vi "Preview_Build.vi"(8 "error in (no error)":errorcluster, 11 "Build in":refnum<class "AB_Build.lvclass">) -> (0 "error out":errorcluster, 1 "GeneratedFiles":path[](array[path]), 3 "Build out":refnum<class "AB_Build.lvclass">, 4 "GeneratedFileGUIDs":string[](array[string]), 5 "OutputDirectory":path)   [LabVIEW 2020, in "AB_Build.lvclass"]
uses:
  <vilib>/AppBuilder/AB_Classes/Build/AB_Build.lvclass
  <vilib>/AppBuilder/AB_Classes/Build/AB_Build.lvclass/AB_Build.ctl
  <vilib>/AppBuilder/AB_Source_Inclusion.ctl
  <resource>/Framework/Providers/Common/provcom_StringGlobals.vi
  <vilib>/AppBuilder/AB_Classes/Destination/AB_Destination.lvclass
  <vilib>/AppBuilder/AB_Classes/Source/AB_Source.lvclass
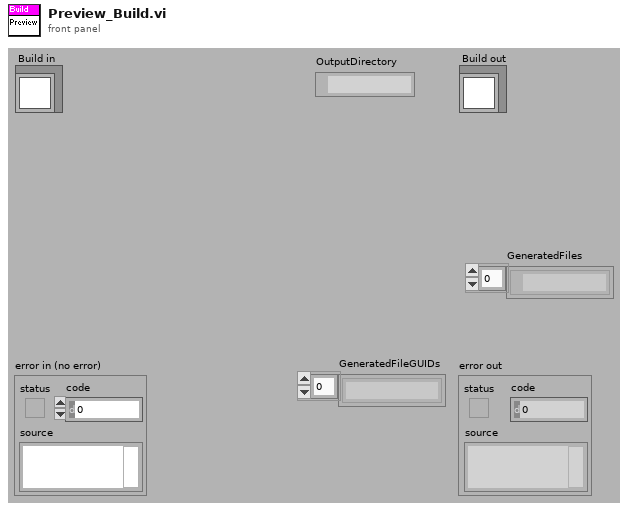
[diagram p1: front panel]
types:
  T1 = typedef "AB_Source_Inclusion.ctl" = enum16{"IncludeIfReferenced", "Include", "Exclude", "TopLevel"}
  T2 = typedef "mxLvBuildError.ctl" = refnum<user-event>
  T3 = typedef "AB_Destination.ctl" = cluster{"destName":string, "path":path, "libraryName":string, "preserveHierarchy":bool, "eng_inBuild":bool, "eng_libraryReference":refnum<vi>, "eng_restictAddToNewLibrary":bool}
  T4 = typedef "AB_Source.ctl" = cluster{"path":path, "itemID":string, "parentIndex":i32, "sourceInclusion":T1, "destinationIndex":i32, "properties":T5[], "newName":string, "lvfile":bool, "valid":bool, "eng_inBuild":bool, "eng_isNonVILink":bool, "Amalgamation":bool, "Amalgamation Piece":bool, "eng_delimitedName":string, "preventRename":bool}
  T5 = typedef "AB_Source_Properties.ctl" = cluster{"sourcePropertyType":T6, "value":variant}
  T6 = typedef "AB_Source_Property_Type.ctl" = enum16{"Remove block diagram", "Remove front panel", "Password", "Window has title bar", "Show menu bar", "Show vertical scroll bar", "Show horizontal scroll bar", "Show toolbar", "Show Abort button", "Show fp when called", "Window behavior", "Allow user to close window", "Window run-time position", "Run when opened", "Allow debugging", "Auto error handling", "Generate guard code", "Use stack variables", "Expression folding", "Integer only", "Inline subVI"}
  T7 = typedef "ItemRef.ctl" = u64
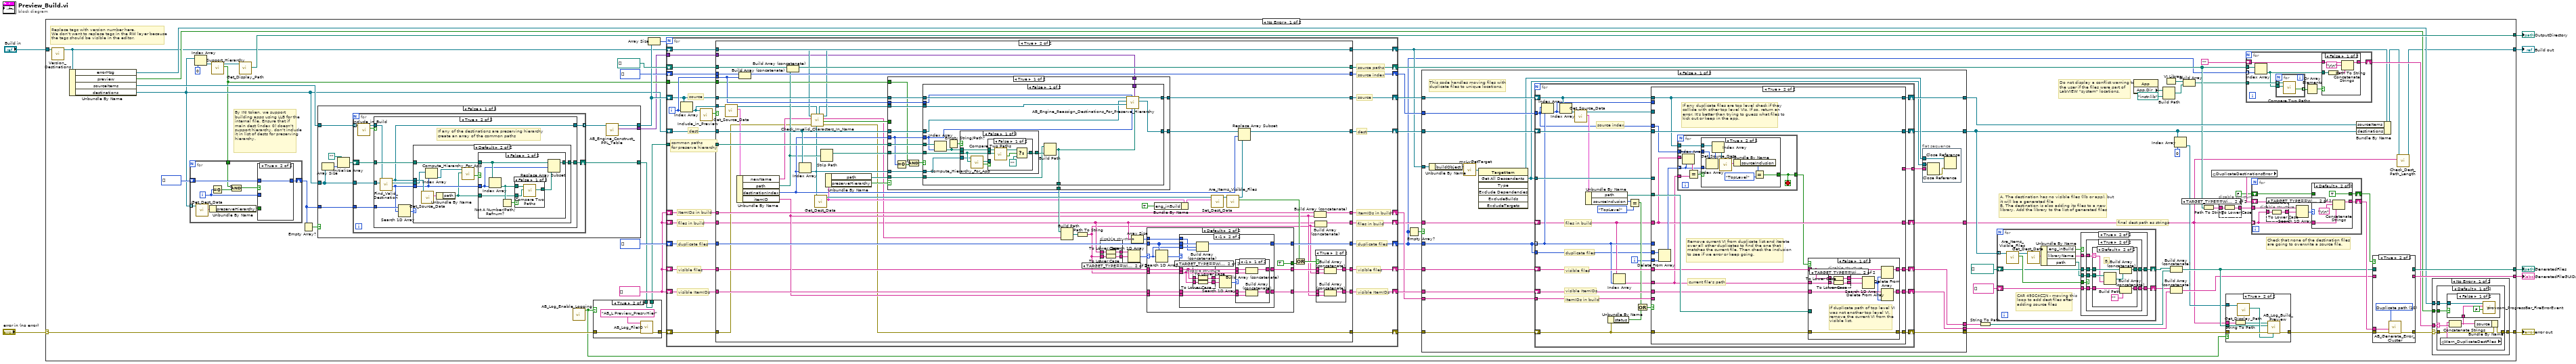
[diagram p0: block diagram]
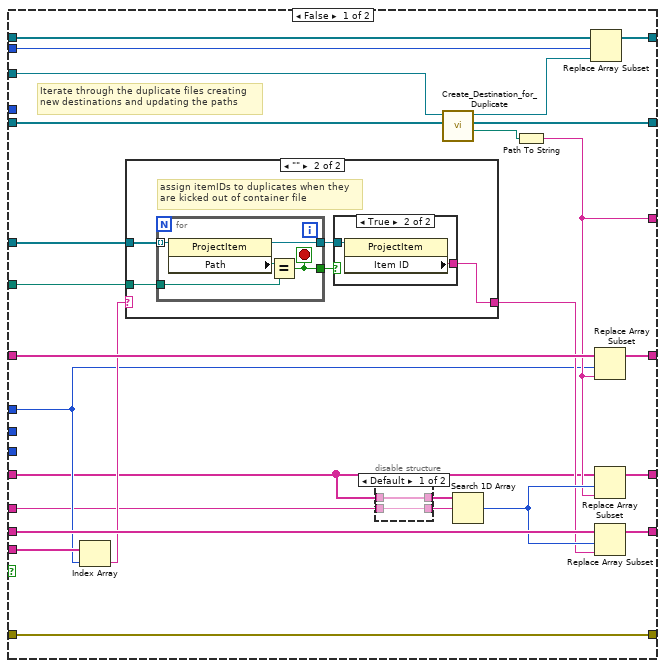
[diagram p3: hidden frame]
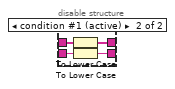
[diagram p4: hidden frame]
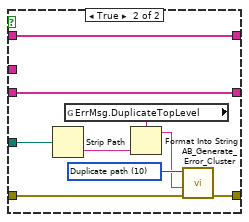
[diagram p9: hidden frame]
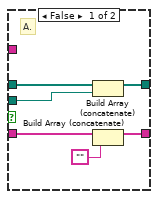
[diagram p13: hidden frame]
diagram:
  n1 = case shown="No Error" "error in (no error)" {
    selector: "error in (no error)" -> [w31 w663]
    tunnel: [w49 w663] -> w6
    tunnel: [w16 w662] -> w4
    tunnel: "Build in" -> [w14 w662]
    tunnel: [w56 _] -> w3
    tunnel: [w55 _] -> w2
    tunnel: [w57 _] -> w1
    frame No Error {
      w37 = string[] []
      # "Replace tags with version number here.\nWe don't want to replace tags in the RW layer because\nthe tags should be visible in the editor."
      # "final dest path as strings"
      # "Do not display a conflict warning to the user if the files were part of LabVIEW \"system\" locations."
      # "By INI token, we support building apps using LLB for the internal file. Ensure that if main dest (index 0) doesn't support hierarchy, don't include it in list of dests for preserving hierarchy."
      # "A. The destination has no visible files (llb or app), but it will be a generated file\nB. The destination is also adding its files to a new library. Add the library to the list of generated files"
      # "Check that none of the destination files are going to overwrite a source file."
      n2 = call <vilib>:"Version_Destinations.vi"("Class in"=w14) -> ("Class out"=w13:refnum<class "AB_Build.lvclass">)  [unwired: 9 in, 1 out]
      n3 = Unbundle By Name(w13) -> ("errorMsg"=w52:T2, "preview"=w50:bool, "sourceItems"=w69:refnum<class "AB_Source.lvclass">[], "destinations"=w35:refnum<class "AB_Destination.lvclass">[])
      n4 = Index Array(array=w35, index=0) -> (element=w34:refnum<class "AB_Destination.lvclass">)
      n5 = call-dynamic "Support_Hierarchy.vi"("AB_Destination in"=w34) -> ("support hierarchy"=w32:bool, "AB_Destination out"=w33:refnum<class "AB_Destination.lvclass">)  [unwired: 1 in, 8 out]
      n6 = for {
        tunnel: w35 -> [w648] mode=indexing
        shift-right: [w650] -> w70
        shift-left: i32[] [] -> [w649]
        tunnel: w32 -> [w645]
        i -> [w647]
        n7 = call <vilib>:"Get_Dest_Data.vi"("Class in"=w648) -> ("destName"=w652:T3)  [unwired: 1 in, 9 out]
        n8 = Unbundle By Name(w652) -> ("preserveHierarchy"=w651:bool)
        n9 = Equal To 0?(x=w647) -> (x = 0?=w646:bool)
        n10 = Compound Arithmetic op=AND(invert w645, w646) -> (w644:bool)
        n11 = case shown="True" w644 {
          tunnel: w651 -> [w656 _]
          tunnel: [w655 w661] -> w650
          tunnel: w649 -> [w654 w661]
          tunnel: w647 -> [w653 _]
          frame False {
            n12 = case shown="False" w656 {
              tunnel: w653 -> [_ w660]
              tunnel: [w657 w659] -> w655
              tunnel: w654 -> [w657 w658]
              frame False {
              }
              frame True {
                n13 = Build Array (concatenate)(w658, w660) -> (w659:i32[])
              }
            }
          }
          frame True {
          }
        }
      }
      n14 = call-dynamic "Get_Display_Path.vi"("AB_Destination in"=w33) -> ("displayPath"=w57:path)  [unwired: 1 in, 9 out]
      n15 = Empty Array?(array=w70) -> (empty?=w71:bool)
      n16 = case shown="False" w71 {
        tunnel: w35 -> [w338 w386]
        tunnel: w69 -> [w341 w388]
        tunnel: w70 -> [w340 _]
        tunnel: [w339 _] -> w29
        tunnel: [w337 w387] -> w68
        tunnel: [w335 _] -> w10
        frame False {
          n17 = Array Size(array=w338) -> (size(s)=w344:i32)
          n18 = Initialize Array(path "", w344) -> (w342:path[])
          n19 = for {
            shift-right: [w351] -> w339
            shift-left: w342 -> [w350]
            tunnel: w341 -> [w347] mode=indexing
            tunnel: w340 -> [w352]
            tunnel: [w348] -> w336 mode=indexing
            tunnel: w338 -> [w349]
            n20 = call-dynamic "Include_in_Build.vi"("AB_Source in"=w347) -> ("includeInBuild"=w345:bool, "AB_Source out"=w346:refnum<class "AB_Source.lvclass">)  [unwired: 1 in, 8 out]
            n21 = case shown="True" w345 {
              tunnel: w352 -> [_ w363]
              tunnel: [w353 w361] -> w351
              tunnel: w350 -> [w353 w360]
              tunnel: w346 -> [w354 w359]
              tunnel: w349 -> [_ w358]
              tunnel: [w354 w356] -> w348
              frame False {
              }
              frame True {
                # "If any of the destinations are preserving hierarchy\ncreate an array of the common paths"
                n22 = call <vilib>:"Find_Valid_Destination.vi"("Destinations in"=w358, "AB_Source in"=w359) -> ("destinationIndex"=w357:i32, "Destinations out"=w355:refnum<class "AB_Destination.lvclass">[], "AB_Source out"=w356:refnum<class "AB_Source.lvclass">)  [unwired: 1 in, 6 out]
                n23 = Search 1D Array(1D array=w363, element=w357) -> (index of element=w362:i32)  [unwired: 1 out]
                n24 = case shown="Default" w362 {
                  tunnel: [w364 w372] -> w361
                  tunnel: w360 -> [w364 w373]
                  tunnel: w357 -> [_ w367]
                  tunnel: w356 -> [_ w370]
                  tunnel: w355 -> [_ w368]
                  frame -1 {
                  }
                  frame Default {
                    n25 = call <vilib>:"Get_Source_Data.vi"("Class in"=w370) -> ("data"=w371:T4)  [unwired: 1 in, 9 out]
                    n26 = Index Array(array=w368, index=w367) -> (element=w366:refnum<class "AB_Destination.lvclass">)
                    n27 = Unbundle By Name(w371) -> ("path"=w365:path)
                    n28 = call-dynamic "Compute_Hierarchy_For_App.vi"("sourcePath"=w365, "AB_Destination in"=w366) -> ("relative to AppDir"=w369:bool)  [unwired: 1 in, 8 out]
                    n29 = case shown="False" w369 {
                      tunnel: w373 -> [w378 w385]
                      tunnel: [w377 w385] -> w372
                      tunnel: w367 -> [w375 _]
                      tunnel: w365 -> [w374 _]
                      frame False {
                        n30 = Index Array(array=w378, index=w375) -> (element=w379:path)
                        n31 = Not A Number/Path/Refnum?(number/path/refnum=w379) -> (NaN/Path/Refnum?=w380:bool)
                        n32 = case shown="False" w380 {
                          tunnel: w379 -> [w383 _]
                          tunnel: w374 -> [w382 w384]
                          tunnel: [w381 w384] -> w376
                          frame False {
                            n33 = call <vilib>:"Compare Two Paths.vi"("Path 2"=w382, "Path 1"=w383) -> ("Common Path"=w381:path)  [unwired: 1 in, 8 out]
                          }
                          frame True {
                          }
                        }
                        n34 = Replace Array Subset(array=w378, new element=w376, index=w375) -> (w377:path[])
                      }
                      frame True {
                        # "If source file path is relative to LabVIEW dir (when dest is an app), don't include LabVIEW's dir in the list of common paths. This reduces the depth of the hierarchy we compute.\nDo standard hierarchy calculations for other dests."
                      }
                    }
                  }
                }
              }
            }
          }
          n35 = call <vilib>:"AB_Engine_Construct_PPL_Table.vi"("sources in"=w336) -> ("PPL Table"=w335:variant, "sources out"=w337:refnum<class "AB_Source.lvclass">[])  [unwired: 8 in, 1 out]
        }
        frame True {
          n36 = for {
            tunnel: w388 -> [w391] mode=indexing
            tunnel: [w392] -> w387 mode=indexing
            tunnel: w386 -> [w393]
            n37 = call-dynamic "Include_in_Build.vi"("AB_Source in"=w391) -> ("includeInBuild"=w389:bool, "AB_Source out"=w390:refnum<class "AB_Source.lvclass">)  [unwired: 1 in, 8 out]
            n38 = case shown="True" w389 {
              tunnel: w390 -> [w394 w397]
              tunnel: w393 -> [_ w396]
              tunnel: [w394 w395] -> w392
              frame False {
              }
              frame True {
                # "Still have to validate destinations to make sure nonVI files aren't targeted into an llb/zip and amalgamation files aren't targeted into an llb"
                n39 = call <vilib>:"Find_Valid_Destination.vi"("Destinations in"=w396, "AB_Source in"=w397) -> ("AB_Source out"=w395:refnum<class "AB_Source.lvclass">)  [unwired: 1 in, 8 out]
              }
            }
          }
        }
      }
      n40 = call <vilib>:"AB_Log_Enable_Logging.vi"() -> ("log?"=w30:bool)  [unwired: 2 in, 9 out]
      n41 = case shown="True" w30 {
        tunnel: w31 -> [w246 w249]
        tunnel: [w246 w248] -> w21
        tunnel: w29 -> [w245 w247]
        tunnel: [w245 w247] -> w28
        frame False {
        }
        frame True {
          n42 = call <vilib>:"AB_Log_FileIO.vi"("error in (no error)"=w249, "newSection"="AB_L Preview_PresrvHier" ("data")) -> ("error out"=w248:errorcluster)  [unwired: 3 in, 6 out]
        }
      }
      n43 = Array Size(array=w68) -> (size(s)=w79:i32)
      n44 = for {
        N: w79 -> [_]
        shift-right: [w431] -> w65
        shift-left: w68 -> [w432]
        shift-right: [w449] -> w47
        shift-left: w37 -> [w450]
        shift-right: [w448] -> w48
        shift-left: w37 -> [w447]
        shift-right: [w445] -> w66
        shift-left: w35 -> [w446]
        shift-right: [w443] -> w27
        shift-left: path[] [] -> [w444]
        tunnel: w28 -> [w442]
        shift-right: [w441] -> w12
        shift-left: i32[] [] -> [w440]
        shift-right: [w438] -> w63
        shift-left: i32[] [] -> [w439]
        shift-right: [w435] -> w60
        shift-left: w37 -> [w436]
        shift-right: [w434] -> w59
        shift-left: w37 -> [w433]
        tunnel: w32 -> [w428]
        shift-right: [w426] -> w20
        shift-left: w21 -> [w427]
        shift-right: [w424] -> _
        shift-left: w13 -> [w425]
        tunnel: w10 -> [w423]
        i -> [w437]
        # "source index"
        # "dest"
        # "source"
        # "dest"
        # "visible ItemIDs"
        # "ItemIDs in build"
        # "visible ItemIDs"
        # "ItemIDs in build"
        # "visible files"
        # "duplicate files"
        # "source paths"
        # "files in build"
        # "visible files"
        # "duplicate files"
        # "common paths\nfor preserve hierarchy"
        # "source"
        # "files in build"
        n45 = Index Array(array=w432, index=w437) -> (element=w429:refnum<class "AB_Source.lvclass">)
        n46 = call-dynamic "Include_in_Preview.vi"("AB_Source in"=w429) -> ("includeInPreview"=w430:bool)  [unwired: 9 in, 1 out]
        n47 = case shown="True" w430 {
          tunnel: w437 -> [_ w486]
          tunnel: w450 -> [w460 w478]
          tunnel: [w460 w505] -> w449
          tunnel: [w461 w520] -> w448
          tunnel: w447 -> [w461 w465]
          tunnel: w429 -> [_ w484]
          tunnel: w446 -> [w459 w492]
          tunnel: [w459 w518] -> w445
          tunnel: w444 -> [w458 w516]
          tunnel: [w458 w487] -> w443
          tunnel: w442 -> [_ w510]
          tunnel: [w457 w507] -> w441
          tunnel: w440 -> [w457 w506]
          tunnel: w439 -> [w456 w499]
          tunnel: [w456 w488] -> w438
          tunnel: w436 -> [w455 w498]
          tunnel: [w455 w494] -> w435
          tunnel: [w454 w497] -> w434
          tunnel: w433 -> [w454 w496]
          tunnel: w432 -> [w453 w490]
          tunnel: [w453 w489] -> w431
          tunnel: w428 -> [_ w477]
          tunnel: w427 -> [w452 w474]
          tunnel: [w452 w473] -> w426
          tunnel: w425 -> [w451 w472]
          tunnel: [w451 w471] -> w424
          tunnel: w423 -> [_ w466]
          frame False {
          }
          frame True {
            n48 = call <vilib>:"Get_Source_Data.vi"("Class in"=w484) -> ("data"=w485:T4, "Class out"=w470:refnum<class "AB_Source.lvclass">)  [unwired: 1 in, 8 out]
            n49 = Unbundle By Name(w485) -> ("newName"=w475:string, "path"=w481:path, "destinationIndex"=w482:i32, "itemID"=w493:string)
            n50 = Build Array (concatenate)(w499, w486) -> (w488:i32[])
            n51 = Build Array (concatenate)(w516, w481) -> (w487:path[])
            n52 = Index Array(array=w492, index=w482) -> (element=w476:refnum<class "AB_Destination.lvclass">)
            n53 = call-dynamic "Check_Invalid_Characters_In_Name.vi"("AB_Destination in"=w476, "AB_Source in"=w470, "error in (no error)"=w474, "file name in"=w475, "Build in"=w472) -> ("error out"=w473:errorcluster, "updated"=w468:bool, "file name out"=w467:string, "Build out"=w471:refnum<class "AB_Build.lvclass">, "AB_Source out"=w469:refnum<class "AB_Source.lvclass">)  [unwired: 1 in, 1 out]
            n54 = call <vilib>:"Get_Dest_Data.vi"("Class in"=w476) -> ("destName"=w483:T3, "Class out"=w513:refnum<class "AB_Destination.lvclass">)  [unwired: 1 in, 8 out]
            n55 = Strip Path(path=w481) -> (stripped path=w509:path)  [unwired: 1 out]
            n56 = Unbundle By Name(w483) -> ("path"=w479:path, "preserveHierarchy"=w511:bool)
            n57 = case shown="True" w511 {
              tunnel: w510 -> [w550 _]
              tunnel: w509 -> [w549 _]
              tunnel: [w547 w590] -> w508
              tunnel: w479 -> [w548 w590]
              tunnel: w482 -> [w539 _]
              tunnel: w492 -> [w546 w591]
              tunnel: [w545 w591] -> w491
              tunnel: w490 -> [w544 w588]
              tunnel: [w543 w587] -> w489
              tunnel: w486 -> [w542 w589]
              tunnel: w469 -> [w541 w586]
              tunnel: w477 -> [w538 _]
              tunnel: w476 -> [w536 _]
              tunnel: w468 -> [_ w585]
              tunnel: w466 -> [w535 _]
              frame True {
                n58 = Equal To 0?(x=w539) -> (x = 0?=w540:bool)
                n59 = Compound Arithmetic op=AND(invert w538, w540) -> (w537:bool)
                n60 = case shown="False" w537 {
                  tunnel: w550 -> [w566 _]
                  tunnel: w549 -> [w564 _]
                  tunnel: w548 -> [w562 w582]
                  tunnel: [w558 w582] -> w547
                  tunnel: w546 -> [w555 w583]
                  tunnel: [w554 w583] -> w545
                  tunnel: w544 -> [w557 w584]
                  tunnel: [w553 w584] -> w543
                  tunnel: w542 -> [w552 _]
                  tunnel: w541 -> [w556 _]
                  tunnel: w539 -> [w559 _]
                  tunnel: w536 -> [w560 _]
                  tunnel: w535 -> [w551 _]
                  frame False {
                    n61 = Index Array(array=w566, index=w559) -> (element=w561:path)
                    n62 = Empty String/Path?(string/path=w561) -> (empty?=w565:bool)
                    n63 = case shown="False" w565 {
                      tunnel: w564 -> [w568 w581]
                      tunnel: w561 -> [w572 _]
                      tunnel: [w571 w580] -> w563
                      tunnel: w560 -> [w567 _]
                      frame False {
                        n64 = call-dynamic "Compute_Hierarchy_For_App.vi"("sourcePath"=w568, "AB_Destination in"=w567) -> ("relative to AppDir"=w570:bool, "destinationPath"=w569:path)  [unwired: 1 in, 7 out]
                        n65 = case shown="False" w570 {
                          tunnel: w568 -> [w578 _]
                          tunnel: w572 -> [w577 _]
                          tunnel: [w573 w579] -> w571
                          tunnel: w569 -> [_ w579]
                          frame False {
                            n66 = call <vilib>:"Compare Two Paths.vi"("Path 2"=w578, "Path 1"=w577) -> ("Path 2 Relative to Path 1?"=w574:bool, "Relative Path from 1 to 2"=w575:path)  [unwired: 1 in, 7 out]
                            n67 = Select(t=w575, s=w574, f=path "") -> (s? t:f=w573:path)
                          }
                          frame True {
                          }
                        }
                      }
                      frame True {
                        n68 = call <vilib>:"AB_Convert_To_Relative_Path.vi"("absolute path"=w581) -> ("relative path"=w580:path)  [unwired: 10 in]
                      }
                    }
                    n69 = Build Path(base path=w562, name or relative path=w563) -> (appended path=w558:path)
                    n70 = call <vilib>:"AB_Engine_Reassign_Destinations_For_Preserve_Hierarchy.vi"("newPath"=w558, "PPL Table"=w551, "parentIndex in"=w559, "source index"=w552, "source"=w556, "destinations in"=w555, "sources in"=w557) -> ("destination out"=w554:refnum<class "AB_Destination.lvclass">[], "sources out"=w553:refnum<class "AB_Source.lvclass">[])  [unwired: 2 in, 1 out]
                  }
                  frame True {
                    # "By INI token, we support building apps using LLB for the internal file. Ensure that if main dest (index 0) doesn't support hierarchy, don't try preserving hierarchy since we can't."
                  }
                }
              }
              frame False {
                n71 = case shown="True" w585 {
                  tunnel: w589 -> [_ w596]
                  tunnel: w588 -> [w592 w595]
                  tunnel: [w592 w594] -> w587
                  tunnel: w586 -> [_ w593]
                  frame False {
                  }
                  frame True {
                    # "If filename was updated, update the value in the source array."
                    n72 = Replace Array Subset(array=w595, new element=w593, index=w596) -> (w594:refnum<class "AB_Source.lvclass">[])
                  }
                }
              }
            }
            n73 = Build Path(base path=w508, name or relative path=w467) -> (appended path=w480:path)
            n74 = Path To String(path=w480) -> (string=w463:string)
            n75 = disable-structure shown="TARGET_TYPE==Windows" {
              disable-tunnel: w465 -> [w522 w525]
              disable-tunnel: [w522 w526] -> w464
              disable-tunnel: w463 -> [w521 w524]
              disable-tunnel: [w521 w523] -> w462
              frame condition #0 {
              }
              frame condition #1 (active) {
                n76 = To Lower Case(string=w525) -> (all lower case string=w526:string[])
                n77 = To Lower Case(string=w524) -> (all lower case string=w523:string)
              }
            }
            n78 = Search 1D Array(1D array=w464, element=w462) -> (index of element=w519:i32)  [unwired: 1 out]
            n79 = Array Size(array=w465) -> (size(s)=w500:i32)
            n80 = case shown="Default" w519 {
              selector: w519 -> [_ w608]
              tunnel: w500 -> [_ w603]
              tunnel: [w599 w611] -> w507
              tunnel: w506 -> [w599 w610]
              tunnel: [_ TRUE] -> w502
              tunnel: w478 -> [w598 w606]
              tunnel: w463 -> [_ w605]
              tunnel: [w598 w604] -> w501
              tunnel: w498 -> [w597 w602]
              tunnel: w493 -> [_ w601]
              tunnel: [w597 w600] -> w495
              frame -1 {
              }
              frame Default {
                n81 = Search 1D Array(1D array=w610, element=w608) -> (index of element=w609:i32)  [unwired: 1 out]
                n82 = case shown="-1" w609 {
                  tunnel: w603 -> [w613 w624]
                  tunnel: [w616 w629] -> w611
                  tunnel: w610 -> [w615 w628]
                  tunnel: w608 -> [_ w627]
                  tunnel: w606 -> [w614 w620]
                  tunnel: w605 -> [_ w618]
                  tunnel: [w614 w625] -> w604
                  tunnel: w602 -> [w612 w623]
                  tunnel: w601 -> [_ w622]
                  tunnel: [w612 w621] -> w600
                  frame Default {
                    n83 = Build Array (concatenate)(w615, w613) -> (w616:i32[])
                  }
                  frame -1 {
                    n84 = disable-structure shown="TARGET_TYPE==Windows" {
                      disable-tunnel: w620 -> [w631 w634]
                      disable-tunnel: [w631 w635] -> w619
                      disable-tunnel: w618 -> [w630 w633]
                      disable-tunnel: [w630 w632] -> w617
                      frame condition #0 {
                      }
                      frame condition #1 (active) {
                        n85 = To Lower Case(string=w634) -> (all lower case string=w635:string[])
                        n86 = To Lower Case(string=w633) -> (all lower case string=w632:string)
                      }
                    }
                    n87 = Build Array (concatenate)(w628, w627, w624) -> (w629:i32[])
                    n88 = Search 1D Array(1D array=w619, element=w617) -> (index of element=w626:i32)  [unwired: 1 out]
                    n89 = case shown="-1" w626 {
                      tunnel: w620 -> [w641 w643]
                      tunnel: w618 -> [w640 _]
                      tunnel: [w639 w643] -> w625
                      tunnel: w623 -> [w638 w642]
                      tunnel: w622 -> [w637 _]
                      tunnel: [w636 w642] -> w621
                      frame -1 {
                        n90 = Build Array (concatenate)(w641, w640) -> (w639:string[])
                        n91 = Build Array (concatenate)(w638, w637) -> (w636:string[])
                      }
                      frame Default {
                      }
                    }
                  }
                }
              }
            }
            n92 = Bundle By Name(cluster=w483, "eng_inBuild"=TRUE) -> (w512:T3)
            n93 = call <vilib>:"Set_Dest_Data.vi"("destName"=w512, "Class in"=w513) -> ("Class out"=w514:refnum<class "AB_Destination.lvclass">)  [unwired: 1 in, 8 out]
            n94 = call-dynamic "Are_Items_Visible_Files.vi"("AB_Destination in"=w514) -> ("itemsVisibleFiles"=w504:bool, "AB_Destination out"=w517:refnum<class "AB_Destination.lvclass">)  [unwired: 1 in, 8 out]
            n95 = Replace Array Subset(array=w491, new element=w517, index=w482) -> (w518:refnum<class "AB_Destination.lvclass">[])
            n96 = Or(x=w504, y=w502) -> (x .or. y?=w503:bool)
            n97 = Build Array (concatenate)(w496, w493) -> (w497:string[])
            n98 = Build Array (concatenate)(w465, w463) -> (w520:string[])
            n99 = case shown="True" w503 {
              tunnel: w501 -> [w528 w534]
              tunnel: [w528 w533] -> w505
              tunnel: w463 -> [_ w532]
              tunnel: w495 -> [w527 w531]
              tunnel: [w527 w530] -> w494
              tunnel: w493 -> [_ w529]
              frame False {
              }
              frame True {
                n100 = Build Array (concatenate)(w534, w532) -> (w533:string[])
                n101 = Build Array (concatenate)(w531, w529) -> (w530:string[])
              }
            }
          }
        }
      }
      n102 = Empty Array?(array=w12) -> (empty?=w11:bool)
      n103 = case shown="False" w11 {
        tunnel: w66 -> [w103 w243]
        tunnel: w65 -> [w102 w244]
        tunnel: w63 -> [w101 _]
        tunnel: [w100 w244] -> w62
        tunnel: w60 -> [w99 w239]
        tunnel: w59 -> [w98 _]
        tunnel: w48 -> [w97 w242]
        tunnel: w47 -> [w96 w241]
        tunnel: [w95 w241] -> w46
        tunnel: [w94 w239] -> w38
        tunnel: [w93 w240] -> w36
        tunnel: w20 -> [w89 w240]
        tunnel: [w88 w243] -> w18
        tunnel: [w87 w242] -> w15
        tunnel: w13 -> [w86 _]
        tunnel: w12 -> [w83 _]
        frame False {
          # "This code handles moving files with duplicate files to unique locations."
          n104 = Unbundle By Name(w86) -> ("buildObject"=w84:T7)
          n105 = call <resource>:"mxLvGetTarget.vi"("Item"=w84) -> ("Target"=w85:refnum<vi>)  [unwired: 1 in, 2 out]
          n106 = invoke class="TargetItem" method="Get All Descendents"(reference=w85) -> (reference out=w91:refnum<vi>, "All Descendents"=w92:refnum<vi>[])  [unwired: 6 in, 5 out]
          n107 = for {
            shift-right: [w132] -> w87
            shift-left: w97 -> [w111]
            shift-right: [w136] -> w88
            shift-left: w103 -> [w135]
            shift-right: [w134] -> w100
            shift-left: w102 -> [w133]
            shift-right: [w131] -> w95
            shift-left: w96 -> [w130]
            tunnel: w83 -> [w112] mode=indexing
            tunnel: w101 -> [w107]
            shift-right: [w128] -> w94
            shift-left: w99 -> [w127]
            tunnel: w98 -> [w126]
            tunnel: w92 -> [w125]
            tunnel: [w122] -> w90
            shift-right: [w121] -> w93
            shift-left: w89 -> [w119]
            tunnel: w83 -> [w108]
            i -> [w109]
            # "duplicate files"
            # "source index"
            # "visible ItemIDs"
            # "visible files"
            # "files in build"
            # "ItemIDs in build"
            n108 = Index Array(array=w107, index=w112) -> (element=w129:i32)
            n109 = Index Array(array=w133, index=w129) -> (element=w124:refnum<class "AB_Source.lvclass">)
            n110 = call <vilib>:"Get_Source_Data.vi"("Class in"=w124) -> ("data"=w120:T4, "Class out"=w123:refnum<class "AB_Source.lvclass">)  [unwired: 1 in, 8 out]
            n111 = Unbundle By Name(w120) -> ("path"=w113:path, "sourceInclusion"=w116:T1)
            n112 = Unbundle By Name(w119) -> ("status"=w117:bool)
            n113 = Index Array(array=w111, index=w112) -> (element=w110:string)
            n114 = Equal?(x=w116, y=AB_Source_Inclusion."TopLevel") -> (x = y?=w114:bool)
            n115 = Or(x=w114, y=w117) -> (x .or. y?=w118:bool)
            n116 = case shown="True" w118 {
              tunnel: [w162 w197] -> w136
              tunnel: w135 -> [w161 w197]
              tunnel: [w160 w186] -> w134
              tunnel: w133 -> [w159 w186]
              tunnel: [w157 w185] -> w132
              tunnel: w111 -> [w156 w185]
              tunnel: [w155 w191] -> w131
              tunnel: w130 -> [w140 w192]
              tunnel: w129 -> [w154 _]
              tunnel: [w153 w190] -> w128
              tunnel: w127 -> [w152 w193]
              tunnel: w126 -> [w151 _]
              tunnel: w112 -> [w142 _]
              tunnel: w125 -> [w148 _]
              tunnel: w123 -> [w147 _]
              tunnel: [w144 _] -> w122
              tunnel: w119 -> [w143 w195]
              tunnel: [w143 w196] -> w121
              tunnel: w113 -> [w141 w194]
              tunnel: w110 -> [w138 w183]
              tunnel: w109 -> [_ w188]
              tunnel: w108 -> [_ w189]
              tunnel: w107 -> [_ w184]
              frame False {
                # "Iterate through the duplicate files creating\nnew destinations and updating the paths"
                n117 = Index Array(array=w151, index=w142) -> (element=w146:string)
                n118 = case shown="\"\"" w146 {
                  selector: w146 -> [w169 _]
                  tunnel: w148 -> [_ w174]
                  tunnel: [w169 w171] -> w145
                  tunnel: w141 -> [_ w170]
                  frame Default {
                  }
                  frame "" {
                    # "assign itemIDs to duplicates when they are kicked out of container file"
                    n119 = for {
                      tunnel: w174 -> [w181] mode=indexing
                      tunnel: w170 -> [w177]
                      tunnel: [w179] -> w172
                      tunnel: [w178] -> w173
                      stop <- w178 stop-if-true
                      n120 = property class="ProjectItem"(reference=w181) -> (reference out=w179:refnum<vi>, "Path"=w180:path)  [unwired: 1 in, 1 out]
                      n121 = Equal?(x=w180, y=w177) -> (x = y?=w178:bool)
                    }
                    n122 = case shown="True" w173 {
                      tunnel: w172 -> [_ w176]
                      tunnel: [_ w175] -> w171
                      frame False {
                      }
                      frame True {
                        n123 = property class="ProjectItem"(reference=w176) -> ("Item ID"=w175:string)  [unwired: 1 in, 2 out]
                      }
                    }
                  }
                }
                n124 = disable-structure shown="Default" {
                  disable-tunnel: w140 -> [w164 w167]
                  disable-tunnel: [w164 w168] -> w139
                  disable-tunnel: w138 -> [w163 w166]
                  disable-tunnel: [w163 w165] -> w137
                  frame condition #0 {
                  }
                  frame condition #1 (active) {
                    n125 = To Lower Case(string=w167) -> (all lower case string=w168:string[])
                    n126 = To Lower Case(string=w166) -> (all lower case string=w165:string)
                  }
                }
                n127 = call-dynamic "Create_Destination_for_Duplicate.vi"("Destinations in"=w161, "AB_Source in"=w147) -> ("newPath"=w149:path, "Destinations out"=w162:refnum<class "AB_Destination.lvclass">[], "AB_Source out"=w158:refnum<class "AB_Source.lvclass">)  [unwired: 2 in, 5 out]
                n128 = Search 1D Array(1D array=w139, element=w137) -> (index of element=w150:i32)  [unwired: 1 out]
                n129 = Path To String(path=w149) -> (string=w144:string)
                n130 = Replace Array Subset(array=w159, new element=w158, index=w154) -> (w160:refnum<class "AB_Source.lvclass">[])
                n131 = Replace Array Subset(array=w156, new element=w144, index=w142) -> (w157:string[])
                n132 = Replace Array Subset(array=w140, new element=w144, index=w150) -> (w155:string[])
                n133 = Replace Array Subset(array=w152, new element=w145, index=w150) -> (w153:string[])
              }
              frame True {
                # "Remove current VI from duplicate list and iterate over all other duplicates to find the one that matches the current file. Then check the inclusion to see if we error or keep going."
                # "current file's path"
                # "If any duplicate files are top level check if they collide with other top level VIs. If so, return an error. It's better than trying to guess what files to kick out or keep in the app."
                n134 = Delete From Array(array=w189, index=w188) -> (array with subset deleted=w187:i32[])  [unwired: 1 in, 1 out]
                n135 = for {
                  tunnel: w187 -> [w200] mode=indexing
                  tunnel: w186 -> [w199]
                  tunnel: w185 -> [w205]
                  tunnel: w184 -> [w204]
                  tunnel: w183 -> [w202]
                  tunnel: [w198] -> w182
                  stop <- w198 stop-if-true
                  n136 = Index Array(array=w205, index=w200) -> (element=w203:string)
                  n137 = Equal?(x=w203, y=w202) -> (x = y?=w201:bool)
                  n138 = case shown="True" w201 {
                    tunnel: w204 -> [_ w214]
                    tunnel: w200 -> [_ w213]
                    tunnel: w199 -> [_ w211]
                    tunnel: [_ w206] -> w198
                    frame False {
                    }
                    frame True {
                      n139 = Index Array(array=w214, index=w213) -> (element=w212:i32)
                      n140 = Index Array(array=w211, index=w212) -> (element=w210:refnum<class "AB_Source.lvclass">)
                      n141 = call <vilib>:"Get_Source_Data.vi"("Class in"=w210) -> ("data"=w209:T4)  [unwired: 1 in, 9 out]
                      n142 = Unbundle By Name(w209) -> ("sourceInclusion"=w208:T1)
                      n143 = Equal?(x=w208, y=AB_Source_Inclusion."TopLevel") -> (x = y?=w206:bool)
                    }
                  }
                }
                n144 = case shown="False" w182 {
                  tunnel: [w223 w238] -> w196
                  tunnel: w195 -> [w223 w237]
                  tunnel: w194 -> [_ w235]
                  tunnel: w193 -> [w221 w230]
                  tunnel: w192 -> [w218 w231]
                  tunnel: [w222 w231] -> w191
                  tunnel: [w220 w230] -> w190
                  tunnel: w183 -> [w216 _]
                  frame False {
                    # "If duplicate path of top level VI was not another top level VI, remove the current VI from the visible list."
                    n145 = disable-structure shown="TARGET_TYPE==Windows" {
                      disable-tunnel: w218 -> [w225 w228]
                      disable-tunnel: [w225 w229] -> w217
                      disable-tunnel: w216 -> [w224 w227]
                      disable-tunnel: [w224 w226] -> w215
                      frame condition #0 {
                      }
                      frame condition #1 (active) {
                        n146 = To Lower Case(string=w228) -> (all lower case string=w229:string[])
                        n147 = To Lower Case(string=w227) -> (all lower case string=w226:string)
                      }
                    }
                    n148 = Search 1D Array(1D array=w217, element=w215) -> (index of element=w219:i32)  [unwired: 1 out]
                    n149 = Delete From Array(array=w218, index=w219) -> (array with subset deleted=w222:string[])  [unwired: 1 in, 1 out]
                    n150 = Delete From Array(array=w221, index=w219) -> (array with subset deleted=w220:string[])  [unwired: 1 in, 1 out]
                  }
                  frame True {
                    w236 = 10 items=["No error", "Argument error", "Memory is full", "Out of zone", "End of file", "File already open", "Generic file I/O error", "File not found", "File permission error", "Disk is full", "Duplicate path", "Too many files open", "System feature not enabled", "Resource file not found", "Cannot add resource", "Resource not found", "Image not found", "Image memory error", "Pen does not exist", "Config type invalid", "Config token not found", "Config parse error", "Config memory error", "Bad external code format", "Bad external code offset", "External code not present", "Null window", "Destroy window error", "Null menu", "Print aborted", "Bad print record", "Print driver error", "Windows error during printing", "Memory error during printing", "Print dialog error", "Generic print error", "Invalid device refnum", "Device not found", "Device parameter error", "Device unit error", "Cannot open device", "Device call aborted", "Generic error", "Cancelled by user", "Object ID too low", "Object ID too high", "Object not in heap", "Unknown heap", "Unknown object (invalid DefProc)", "Unknown object (DefProc not in table)", "Message out of range", "Invalid (null) method", "Unknown message", "Manager call not supported", "Bad address", "Network operation in progress", "Network operation timed out", "Connection is busy", "Network attribute not supported", "Network error", "Address in use", "System out of memory", "Connection aborted", "Connection refused", "Not connected", "Already connected", "Connection closed", "Initialization error (interapplication manager)", "Bad occurrence", "Wait on unbound occurrence handler", "Occurrence queue overflow", "Datalog type conflict", "Unused", "Unrecognized type (interapplication manager)", "Memory corrupt", "Failed to make temporary DLL", "Old CIN version", "Drag socket not found", "Failed to load drop-object", "Failed to register OLE object", "Failed to release OLE object", "Format specifier type mismatch", "Unknown format specifier", "Too few format specifiers", "Too many format specifiers", "Scan failed", "Newer CIN version", "Error converting to variant", "Runtime menu error", "Password tampered", "Variant attribute not found", "Incompatible variant data type", "Event data is not available", "Event Store is not present", "Occurrence is not found", "Event Queue is not created", "Event info is not available in the type library", "Refnum passed is NULL", "Error retrieving Class GUID", "Error retrieving CoClass GUID", "Error retrieving TypeLib GUID.", "Bad built application magic bytes.", "Specific driver is different from the specific driver associated with the Logical Name.", "There is no session opened to the class driver.", "Max Error", "MAX - Error with config objects", "MAX - Error loading configuration", "MAX - Group not supported", "Singlecast connections can not send to multicast addresses.", "Multicast connections can not send to singlecast addresses.", "Specified IP address not in multicast address range.", "Attempt to write to read-only multicast connection.", "Attempt to read from write-only multicast connection.", "The buffer used to receive a datagram was smaller than the datagram itself"] ("Code")
                    n151 = Strip Path(path=w235) -> (name=w233:string)  [unwired: 1 out]
                    n152 = global read "provcom_StringGlobals.vi" "ErrMsg.DuplicateTopLevel"() -> (w234:string)
                    n153 = Format Into String(format string=w234, w233) -> (resulting string=w232:string)  [unwired: 2 in, 1 out]
                    n154 = call <vilib>:"AB_Generate_Error_Cluster.vi"("error in (no error)"=w237, "Additional Message"=w232, "Code"=w236) -> ("error out"=w238:errorcluster)  [unwired: 1 in, 7 out]
                  }
                }
              }
            }
          }
          n155 = flat-sequence {
            tunnel: w92 -> [w106]
            tunnel: w91 -> [w105]
            tunnel: w90 -> [_]
            frame #0 {
              n156 = Close Reference(reference=w106) -> (error out=w104:errorcluster)  [unwired: 1 in]
              n157 = Close Reference(reference=w105, error in (no error)=w104) -> ()  [unwired: 1 out]
            }
          }
        }
        frame True {
        }
      }
      n158 = String To Path(string=w46) -> (path=w45:path[])
      n159 = for {
        tunnel: w18 -> [w261] mode=indexing
        shift-right: [w258] -> w44
        shift-left: path[] [] -> [w259]
        shift-right: [w253] -> w40
        shift-left: string[] [] -> [w252]
        # "CAR 49SC4CZN - moving this loop to add dest files after adding source files"
        n160 = call-dynamic "Are_Items_Visible_Files.vi"("AB_Destination in"=w261) -> ("itemsVisibleFiles"=w260:bool, "AB_Destination out"=w256:refnum<class "AB_Destination.lvclass">)  [unwired: 1 in, 8 out]
        n161 = call <vilib>:"Get_Dest_Data.vi"("Class in"=w256) -> ("destName"=w257:T3)  [unwired: 1 in, 9 out]
        n162 = Unbundle By Name(w257) -> ("eng_inBuild"=w251:bool, "libraryName"=w255:string, "path"=w254:path)
        n163 = case shown="True" w251 {
          tunnel: w260 -> [_ w270]
          tunnel: w259 -> [w263 w269]
          tunnel: [w263 w268] -> w258
          tunnel: w255 -> [_ w267]
          tunnel: w254 -> [_ w266]
          tunnel: [w262 w265] -> w253
          tunnel: w252 -> [w262 w264]
          frame False {
            # "Dest not participating in build"
          }
          frame True {
            n164 = case shown="True" w270 {
              tunnel: w269 -> [w276 w282]
              tunnel: [w275 w281] -> w268
              tunnel: w266 -> [w274 w279]
              tunnel: w267 -> [_ w280]
              tunnel: [w271 w278] -> w265
              tunnel: w264 -> [w272 w277]
              frame False {
                # "A."
                n165 = Build Array (concatenate)(w276, w274) -> (w275:path[])
                n166 = Build Array (concatenate)(w272, "") -> (w271:string[])
              }
              frame True {
                n167 = case shown="Default" w280 {
                  selector: w280 -> [_ w289]
                  tunnel: w282 -> [w284 w292]
                  tunnel: [w284 w291] -> w281
                  tunnel: w279 -> [_ w290]
                  tunnel: [w283 w286] -> w278
                  tunnel: w277 -> [w283 w285]
                  frame "" {
                  }
                  frame Default {
                    # "B."
                    n168 = Build Path(base path=w290, name or relative path=w289) -> (appended path=w288:path)
                    n169 = Build Array (concatenate)(w292, w288) -> (w291:path[])
                    n170 = Build Array (concatenate)(w285, "") -> (w286:string[])
                  }
                }
              }
            }
          }
        }
      }
      n171 = property class="App"() -> ("App.Dir"=w24:path)  [unwired: 2 in, 2 out]
      n172 = Build Path(base path=w24, name or relative path=path "instr.lib") -> (appended path=w23:path)
      n173 = VI Library() -> (path=w25:path)
      n174 = Build Array (concatenate)(w44, w45) -> (w43:path[])
      n175 = Build Array (concatenate)(w40, w38) -> (w39:string[])
      n176 = Index Array(array=w18, index=0) -> (element=w19:refnum<class "AB_Destination.lvclass">)
      n177 = Build Array(w25, w23) -> (w26:path[])
      n178 = Path To String(path=w27) -> (string=w9:string[])
      n179 = global read "provcom_StringGlobals.vi" "DuplicateDestinationsError"() -> (w77:string)
      n180 = disable-structure shown="TARGET_TYPE==Windows" {
        disable-tunnel: w9 -> [w80 w81]
        disable-tunnel: [w80 w82] -> w8
        frame condition #0 {
        }
        frame condition #1 (active) {
          n181 = To Lower Case(string=w81) -> (all lower case string=w82:string[])
        }
      }
      n182 = case shown="True" w30 {
        tunnel: w19 -> [_ w334]
        tunnel: w36 -> [w327 w333]
        tunnel: [w327 w332] -> w73
        tunnel: w15 -> [_ w329]
        tunnel: w43 -> [_ w330]
        frame False {
        }
        frame True {
          n183 = String To Path(string=w329) -> (path=w328:path[])
          n184 = call-dynamic "Get_Display_Path.vi"("AB_Destination in"=w334) -> ("displayPath"=w331:path)  [unwired: 1 in, 9 out]
          n185 = call <vilib>:"AB_Log_Build_Preview.vi"("destination path"=w331, "error in (no error)"=w333, "Visible files"=w330, "All files"=w328) -> ("error out"=w332:errorcluster)  [unwired: 7 out]
        }
      }
      n186 = for {
        tunnel: w27 -> [w317]
        tunnel: w12 -> [w316] mode=indexing
        shift-right: [w315] -> w53
        shift-left: "" -> [w314]
        tunnel: w26 -> [w313]
        n187 = Index Array(array=w317, index=w316) -> (element=w311:path)
        n188 = for {
          tunnel: w313 -> [w320] mode=indexing
          tunnel: [w319] -> w312 mode=indexing
          tunnel: w311 -> [w318]
          n189 = call <vilib>:"Compare Two Paths.vi"("Path 2"=w318, "Path 1"=w320) -> ("Path 2 Relative to Path 1?"=w319:bool)  [unwired: 1 in, 8 out]
        }
        n190 = Or Array Elements(Boolean array=w312) -> (logical OR=w310:bool)
        n191 = case shown="False" w310 {
          tunnel: [w325 w326] -> w315
          tunnel: w314 -> [w324 w326]
          tunnel: w311 -> [w322 _]
          frame False {
            n192 = Path To String(path=w322) -> (string=w321:string)
            n193 = Concatenate Strings(w324, "\r\n", w321) -> (w325:string)
          }
          frame True {
          }
        }
      }
      n194 = for {
        tunnel: w8 -> [w412]
        tunnel: w15 -> [w406] mode=indexing
        shift-right: [w408] -> w74
        shift-left: w77 -> [w407]
        shift-right: [w410] -> w75
        shift-left: FALSE -> [w409]
        n195 = disable-structure shown="TARGET_TYPE==Windows" {
          disable-tunnel: w406 -> [w413 w414]
          disable-tunnel: [w413 w415] -> w405
          frame condition #0 {
          }
          frame condition #1 (active) {
            n196 = To Lower Case(string=w414) -> (all lower case string=w415:string)
          }
        }
        n197 = Search 1D Array(1D array=w412, element=w405) -> (index of element=w411:i32)  [unwired: 1 out]
        n198 = case shown="Default" w411 {
          tunnel: [w417 TRUE] -> w410
          tunnel: w409 -> [w417 _]
          tunnel: [w416 w420] -> w408
          tunnel: w407 -> [w416 w421]
          tunnel: w406 -> [_ w418]
          frame -1 {
          }
          frame Default {
            n199 = Concatenate Strings(w421, "\r\n", w418) -> (w420:string)
          }
        }
      }
      n200 = Bundle By Name(cluster=w13, "sourceItems"=w62, "destinations"=w18) -> (w17:refnum<class "AB_Build.lvclass">)
      n201 = case shown="True" w75 {
        tunnel: w73 -> [w400 w404]
        tunnel: [w400 w403] -> w51
        tunnel: w74 -> [_ w402]
        tunnel: [w399 _] -> w56
        tunnel: w43 -> [w399 _]
        tunnel: [w398 _] -> w55
        tunnel: w39 -> [w398 _]
        frame False {
        }
        frame True {
          w401 = 10 items=["No error", "Argument error", "Memory is full", "Out of zone", "End of file", "File already open", "Generic file I/O error", "File not found", "File permission error", "Disk is full", "Duplicate path", "Too many files open", "System feature not enabled", "Resource file not found", "Cannot add resource", "Resource not found", "Image not found", "Image memory error", "Pen does not exist", "Config type invalid", "Config token not found", "Config parse error", "Config memory error", "Bad external code format", "Bad external code offset", "External code not present", "Null window", "Destroy window error", "Null menu", "Print aborted", "Bad print record", "Print driver error", "Windows error during printing", "Memory error during printing", "Print dialog error", "Generic print error", "Invalid device refnum", "Device not found", "Device parameter error", "Device unit error", "Cannot open device", "Device call aborted", "Generic error", "Cancelled by user", "Object ID too low", "Object ID too high", "Object not in heap", "Unknown heap", "Unknown object (invalid DefProc)", "Unknown object (DefProc not in table)", "Message out of range", "Invalid (null) method", "Unknown message", "Manager call not supported", "Bad address", "Network operation in progress", "Network operation timed out", "Connection is busy", "Network attribute not supported", "Network error", "Address in use", "System out of memory", "Connection aborted", "Connection refused", "Not connected", "Already connected", "Connection closed", "Initialization error (interapplication manager)", "Bad occurrence", "Wait on unbound occurrence handler", "Occurrence queue overflow", "Datalog type conflict", "Unused", "Unrecognized type (interapplication manager)", "Memory corrupt", "Failed to make temporary DLL", "Old CIN version", "Drag socket not found", "Failed to load drop-object", "Failed to register OLE object", "Failed to release OLE object", "Format specifier type mismatch", "Unknown format specifier", "Too few format specifiers", "Too many format specifiers", "Scan failed", "Newer CIN version", "Error converting to variant", "Runtime menu error", "Password tampered", "Variant attribute not found", "Incompatible variant data type", "Event data is not available", "Event Store is not present", "Occurrence is not found", "Event Queue is not created", "Event info is not available in the type library", "Refnum passed is NULL", "Error retrieving Class GUID", "Error retrieving CoClass GUID", "Error retrieving TypeLib GUID.", "Bad built application magic bytes.", "Specific driver is different from the specific driver associated with the Logical Name.", "There is no session opened to the class driver.", "Max Error", "MAX - Error with config objects", "MAX - Error loading configuration", "MAX - Group not supported", "Singlecast connections can not send to multicast addresses.", "Multicast connections can not send to singlecast addresses.", "Specified IP address not in multicast address range.", "Attempt to write to read-only multicast connection.", "Attempt to read from write-only multicast connection.", "The buffer used to receive a datagram was smaller than the datagram itself"] ("Code")
          n202 = call <vilib>:"AB_Generate_Error_Cluster.vi"("error in (no error)"=w404, "Additional Message"=w402, "Code"=w401) -> ("error out"=w403:errorcluster)  [unwired: 1 in, 7 out]
        }
      }
      n203 = call-dynamic "Check_Dest_Path_Length.vi"("file build destinations"=w15, "Build in"=w17) -> ("Build out"=w16:refnum<class "AB_Build.lvclass">)  [unwired: 8 in, 1 out]
      n204 = case shown="No Error" w51 {
        selector: w51 -> [w294 w309]
        tunnel: w53 -> [w297 _]
        tunnel: w52 -> [w296 _]
        tunnel: w50 -> [w295 _]
        tunnel: [w293 w309] -> w49
        frame No Error {
          n205 = case shown="Default" w297 {
            selector: w297 -> [w303 _]
            tunnel: w296 -> [w304 _]
            tunnel: w295 -> [w301 _]
            tunnel: w294 -> [w300 w308]
            tunnel: [w298 w308] -> w293
            frame Default {
              n206 = global read "provcom_StringGlobals.vi" "Warn_DuplicateDestFiles"() -> (w302:string)
              n207 = Concatenate Strings(w302, w303) -> (w299:string)
              n208 = case shown="False" w301 {
                tunnel: w304 -> [w307 _]
                tunnel: w299 -> [w306 _]
                frame False {
                  n209 = call <resource>:"provcom_ProgressBar_FireErrorEvent.vi"("Error?"=FALSE, "ErrorText"=w306, "Error event"=w307) -> ()  [unwired: 8 in, 1 out]
                }
                frame True {
                }
              }
              n210 = Bundle By Name(cluster=w300, "source"=w299) -> (w298:errorcluster)
            }
            frame "" {
            }
          }
        }
        frame Error {
        }
      }
    }
    frame Error {
    }
  }
  "error out" <- w6
  "Build out" <- w4
  "GeneratedFiles" <- w3
  "GeneratedFileGUIDs" <- w2
  "OutputDirectory" <- w1
